vi "FIFO.vi"(5 "启用":bool, 7 "元素大小":u32, 11 "数值":dbl) -> (3 "数组":dbl[](array[numeric]))   [LabVIEW 2016, in "多参数状态显示.xctl"]
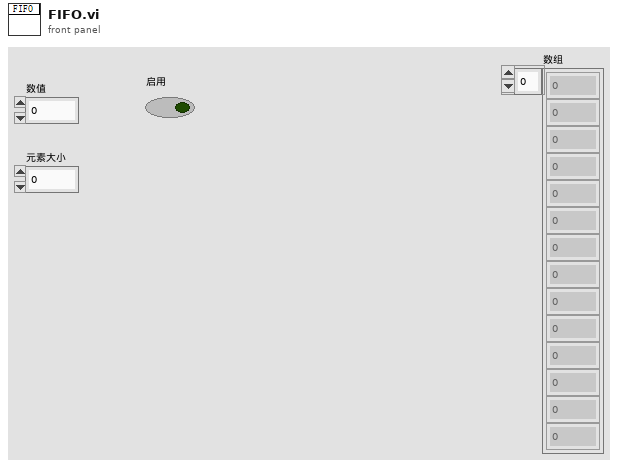
[diagram p1: front panel]
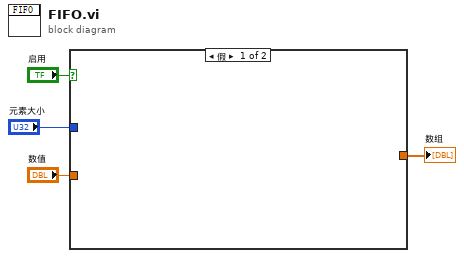
[diagram p0: block diagram]
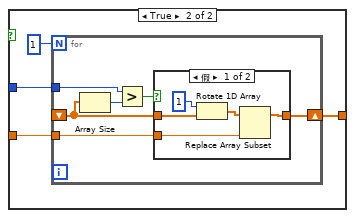
[diagram p2: hidden frame]
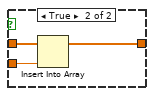
[diagram p3: hidden frame]
diagram:
  n1 = case shown="假" "启用" {
    tunnel: "数值" -> [_ w8]
    tunnel: "元素大小" -> [_ w6]
    tunnel: [_ w5] -> w2
    frame False {
    }
    frame True {
      n2 = for {
        N: 1 -> [_]
        tunnel: w8 -> [w14]
        shift-right: [w13] -> w5
        shift-left: _ -> [w12]
        tunnel: w6 -> [w11]
        n3 = Array Size(array=w12) -> (size(s)=w10:i32)
        n4 = Greater?(x=w11, y=w10) -> (0:w9:bool)
        n5 = case shown="假" w9 {
          tunnel: w14 -> [w18 w22]
          tunnel: [w16 w21] -> w13
          tunnel: w12 -> [w19 w20]
          frame False {
            n6 = Rotate 1D Array(1:w19, 2:1 ("n")) -> (0:w17:dbl[])
            n7 = Replace Array Subset(array=w17, new element=w18) -> (w16:dbl[])  [unwired: 1 in]
          }
          frame True {
            n8 = Insert Into Array(array=w20, new element=w22) -> (w21:dbl[])  [unwired: 1 in]
          }
        }
      }
    }
  }
  "数组" <- w2
